vi "getLeapSecondCount.vi"(10 "UTC Epoch Time":i64=2272060800) -> (2 "Leap Seconds":i64=2272060800)   [LabVIEW 2013, in "Epoch.lvclass"]
doc: "Leap Seconds are defined with reference to Atominc International Time (TAI)"
uses:
  Epoch.lvclass
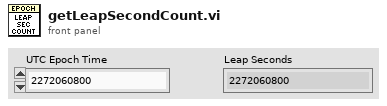
[diagram p1: front panel]
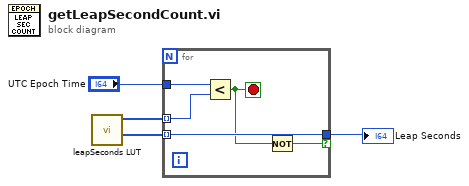
[diagram p0: block diagram]
diagram:
  n1 = call "leapSeconds LUT.vi"() -> ("Leap Seconds"=w2:i64[], "UTC Time"=w4:i64[])  [unwired: 10 in]
  n2 = for {
    tunnel: w4 -> [w9] mode=indexing
    tunnel: "UTC Epoch Time" -> [w8]
    tunnel: w2 -> [w7] mode=indexing
    tunnel: [w7] -> w1 if=w5
    stop <- w6 stop-if-true
    n3 = Less?(x=w8, y=w9) -> (x < y?=w6:bool)
    n4 = Not(x=w6) -> (.not. x?=w5:bool)
  }
  "Leap Seconds" <- w1
